vi "8XY2.vi"(11 "Variables and Memory in":T1 {"GFX" format="%02x"}) -> (3 "Variables and Memory out":T1 {"GFX" format="%02x"})   [LabVIEW 2021]
uses:
  Controls/ClusterF.ctl
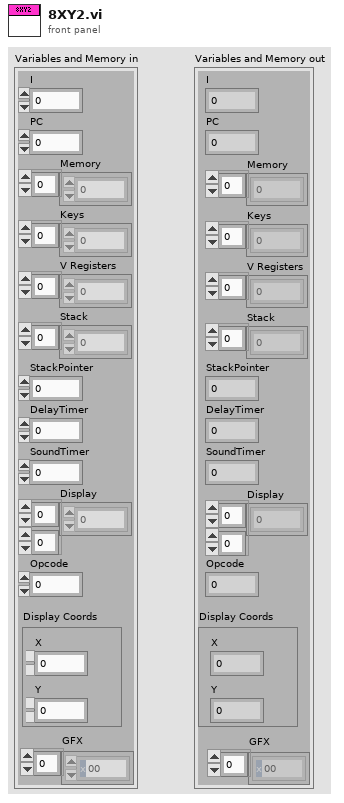
[diagram p1: front panel]
types:
  T1 = typedef "ClusterF.ctl" = cluster{"I":u16, "PC":u16, "Memory":u8[], "Keys":u8[], "V Registers":u8[], "Stack":u16[], "StackPointer":u16, "DelayTimer":u8, "SoundTimer":u8, "Display":u8[][], "Opcode":u16, "Display Coords":cluster{"X":u8, "Y":u8}, "GFX":u8[]}
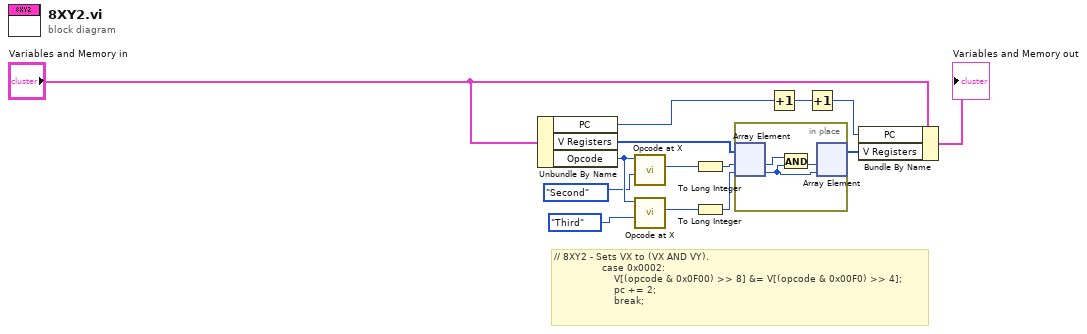
[diagram p0: block diagram]
diagram:
  # "// 8XY2 - Sets VX to (VX AND VY).\n                case 0x0002:\n                    V[(opcode & 0x0F00) >> 8] &= V[(opcode & 0x00F0) >> 4];\n                    pc += 2;\n                    break;"
  n1 = Unbundle By Name("Variables and Memory in") -> ("PC"=w2:u16, "V Registers"=w7:u8[], "Opcode"=w14:u16)
  n2 = call "Opcode at X.vi"("X Position"=enum16{"First", "Second", "Third", "Fourth"}."Second", "Opcode"=w14) -> ("Opcode at X Position (U8)"=w8:u8)  [unwired: 9 in]
  n3 = call "Opcode at X.vi"("X Position"=enum16{"First", "Second", "Third", "Fourth"}."Third", "Opcode"=w14) -> ("Opcode at X Position (U8)"=w6:u8)  [unwired: 9 in]
  n4 = To Long Integer(number=w8) -> (32bit integer=w9:i32)
  n5 = To Long Integer(number=w6) -> (32bit integer=w13:i32)
  n6 = in-place {
    n7 = in-place-array #1(w7, w9, w13) -> (w17:u8, w15:u8)
    n8 = And(x=w17, y=w15) -> (x .and. y?=w16:u8)
    n9 = in-place-array #1(w16, w15) -> (w10:u8[])  [unwired: 2 out]
  }
  n10 = Increment(x=w2) -> (x+1=w1:u16)
  n11 = Increment(x=w1) -> (x+1=w3:u16)
  n12 = Bundle By Name(cluster="Variables and Memory in", "PC"=w3, "V Registers"=w10) -> (→"Variables and Memory out":T1)
